vi "Graph ERD Read List_v1.35.vi"(11 "ERD Graph Cntrl":T2 {"ERD 1"."Scaler" min=1; "ERD 1"."ERD #" format="%.0x"; "ERD 2"."Scaler" min=1; "ERD 2"."ERD #" format="%.0x"; "ERD 3"."Scaler" min=1; "ERD 3"."ERD #" format="%.0x"}) -> (3 "Array":T1[](array[typedef]) {"ERD Number" format="%.0x"})   [LabVIEW 2014]
uses:
  type defs/ERD_Graph_All.ctl
  type defs/ERD_Graph.ctl
  Common/LabVIEW GEA2 Toolkit/LabVIEW_GEA2_Toolkit.lvlibp/type defs/ERD Read Data In.ctl
  Common/LabVIEW GEA2 Toolkit/LabVIEW_GEA2_Toolkit.lvlibp
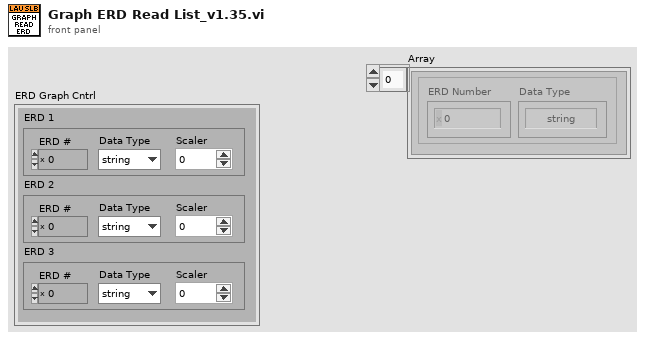
[diagram p1: front panel]
types:
  T1 = typedef "LabVIEW_GEA2_Toolkit.lvlibp/ERD Read Data In.ctl" = cluster{"ERD Number":u16, "Data Type":enum16{"string", "boolean", "uint8_t", "uint16_t", "uint32_t", "uint64_t"}}
  T2 = typedef "ERD_Graph_All.ctl" = cluster{"ERD 3":T3, "ERD 2":T3, "ERD 1":T3}
  T3 = typedef "ERD_Graph.ctl" = cluster{"ERD #":u16, "Scaler":u32, "Data Type":enum16{"string", "boolean", "uint8_t", "uint16_t", "uint32_t"}}
  T4 = enum16{"string", "boolean", "uint8_t", "uint16_t", "uint32_t"}
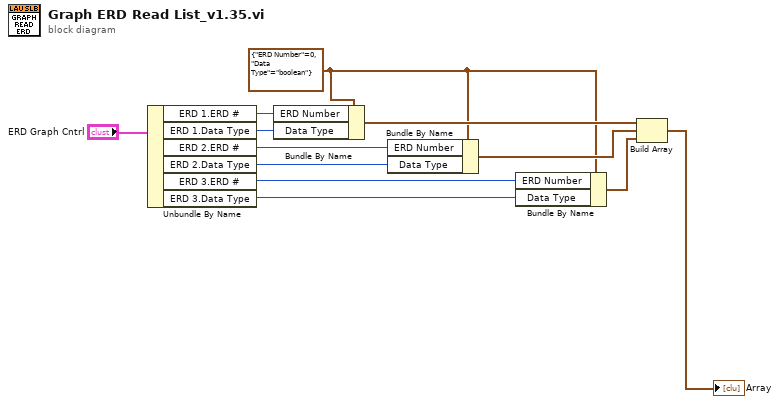
[diagram p0: block diagram]
diagram:
  w7 = T1 {"ERD Number"=0, "Data Type"=enum."boolean"} ("ERD Read Data In 2")
  n1 = Unbundle By Name("ERD Graph Cntrl") -> ("ERD 1.ERD #"=w1:u16, "ERD 1.Data Type"=w2:T4, "ERD 2.ERD #"=w3:u16, "ERD 2.Data Type"=w4:T4, "ERD 3.ERD #"=w5:u16, "ERD 3.Data Type"=w6:T4)
  n2 = Bundle By Name(cluster=w7, "ERD Number"=w1, "Data Type"=w2) -> (w8:T1)
  n3 = Bundle By Name(cluster=w7, "ERD Number"=w3, "Data Type"=w4) -> (w9:T1)
  n4 = Bundle By Name(cluster=w7, "ERD Number"=w5, "Data Type"=w6) -> (w10:T1)
  n5 = Build Array(w8, w9, w10) -> (→"Array":T1[])
